vi "ReadInputDevices.vi"(8 "error in (no error)":errorcluster, 11 "VISA Refnum in":refnum<visa-resource-name>) -> (0 "error out":errorcluster, 1 "hand Brake":bool, 2 "Reverse":bool, 3 "VISA Refnum out":refnum<visa-resource-name>, 4 "Brake":i32, 5 "Throtle":i32, 7 "Steering Wheel":i32)   [LabVIEW 2019]
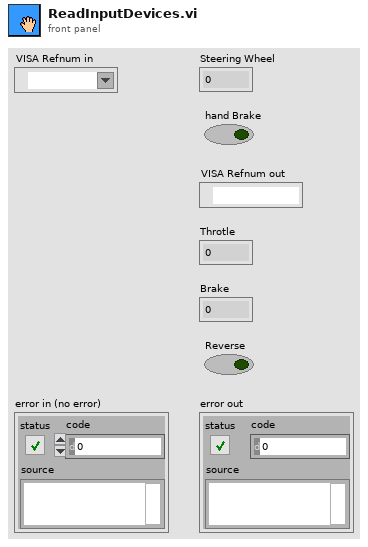
[diagram p1: front panel]
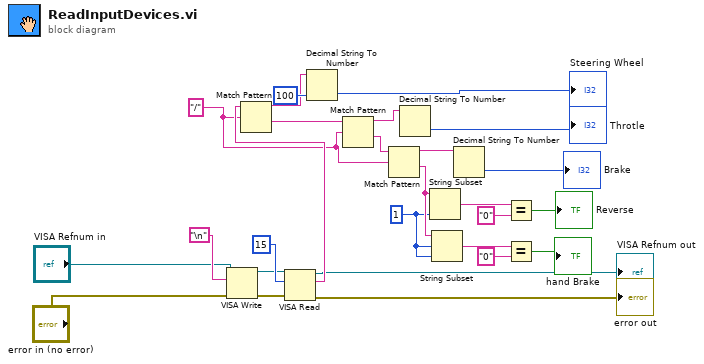
[diagram p0: block diagram]
diagram:
  w19 = 1 ("length (rest)")
  w7 = "/" ("regular expression")
  n1 = VISA Write(VISA resource name="VISA Refnum in", write buffer="\n", error in (no error)="error in (no error)") -> (VISA resource name out=w3:refnum<visa-resource-name>, error out=w4:errorcluster)  [unwired: 1 out]
  n2 = VISA Read(VISA resource name=w3, byte count=u32 15, error in (no error)=w4) -> (VISA resource name out=→"VISA Refnum out":refnum<visa-resource-name>, read buffer=w16:string, error out=→"error out":errorcluster)  [unwired: 1 out]
  n3 = Match Pattern(string=w16, regular expression=w7) -> (before substring=w8:string, after substring=w5:string)  [unwired: 1 in, 2 out]
  n4 = Decimal String To Number(string=w8, default (0L)=100 ("default (0 I32)")) -> (number=→"Steering Wheel":i32)  [unwired: 1 in, 1 out]
  n5 = Match Pattern(string=w5, regular expression=w7) -> (before substring=w10:string, after substring=w6:string)  [unwired: 1 in, 2 out]
  n6 = Match Pattern(string=w6, regular expression=w7) -> (before substring=w12:string, after substring=w20:string)  [unwired: 1 in, 2 out]
  n7 = Decimal String To Number(string=w10) -> (number=→"Throtle":i32)  [unwired: 2 in, 1 out]
  n8 = String Subset(string=w20, length (rest)=w19) -> (substring=w25:string)  [unwired: 1 in]
  n9 = String Subset(string=w20, offset (0)=w19, length (rest)=w19) -> (substring=w21:string)
  n10 = Decimal String To Number(string=w12) -> (number=→"Brake":i32)  [unwired: 2 in, 1 out]
  n11 = Equal?(x=w25, y="0") -> (x = y?=→"Reverse":bool)
  n12 = Equal?(x=w21, y="0") -> (x = y?=→"hand Brake":bool)
